vi "Get Slewing Test Settings.vi"(11 "Model in":refnum<class "Model.lvclass">) -> (2 "Slewing Test Settings":T1 {"Settling Time (s)" format="%.4g"; "Hold Time (s)" format="%.4g"; "Ramp Time (s)" format="%.4g"; "Max Instance Force Error (N)" format="%.4g"; "Amplitude (N)" format="%.4g"; "Max Moment (NM)" format="%.4f"; "Max Force Error (N)" format="%.4f"}, 3 "Model out":refnum<class "Model.lvclass">)   [LabVIEW 2016]
uses:
  Model.lvclass
  Typedefs/SlewingTestSettings.ctl
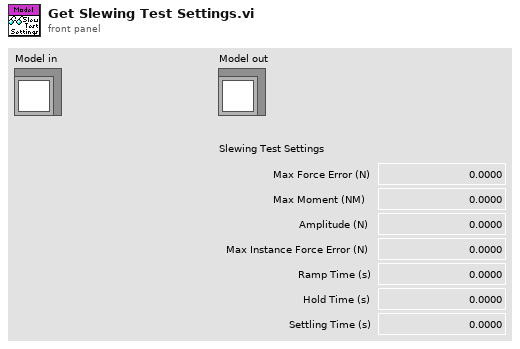
[diagram p1: front panel]
types:
  T1 = typedef "SlewingTestSettings.ctl" = cluster{"Max Force Error (N)":dbl, "Max Moment (NM)":dbl, "Amplitude (N)":dbl, "Max Instance Force Error (N)":dbl, "Ramp Time (s)":dbl, "Hold Time (s)":dbl, "Settling Time (s)":dbl}
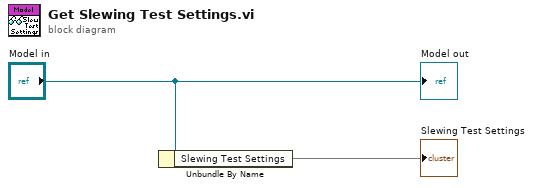
[diagram p0: block diagram]
diagram:
  n1 = Unbundle By Name("Model in") -> ("Slewing Test Settings"=→"Slewing Test Settings")
  "Model out" <- "Model in"
